vi "DAQ1.vi"() -> ()   [LabVIEW 2015]
panel:
  out "size(s)":i32
  out "Y":dbl[](array[numeric])
  out "dt":dbl
  out "t0":timestamp
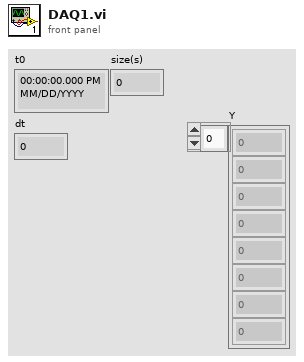
[diagram p1: front panel]
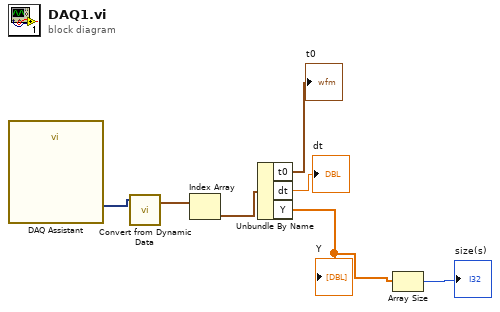
[diagram p0: block diagram]
diagram:
  n1 = call "DAQ Assistant"() -> ("data"=w7:dynamicdata)  [unwired: 17 in, 2 out]
  n2 = call "Convert from Dynamic Data"("Dynamic Data Type"=w7) -> ("Array of Waveform"=w6:waveform(dbl)[])  [unwired: 3 in]
  n3 = Index Array(array=w6) -> (element=w5:waveform(dbl))  [unwired: 1 in]
  n4 = Unbundle By Name(w5) -> ("t0"=→"t0":timestamp, "dt"=→"dt":dbl, "Y"=w2:dbl[])
  "Y" <- w2
  n5 = Array Size(array=w2) -> (size(s)=→"size(s)":i32)
